vi "Pololu.Mgr - Get Status.vi"(8 "error in (no error)":errorcluster, 11 "PololuCtrl in":refnum<class "PololuCtrl.lvclass">) -> (0 "error out":errorcluster, 1 "Pos(Deg)":dbl[](array[numeric]), 2 "Moving":bool, 3 "PololuCtrl out":refnum<class "PololuCtrl.lvclass">)   [LabVIEW 2018, in "PololuCtrl.lvclass"]
uses:
  PololuCtrl.lvclass
  SubVIs/Pololu.Commands.ctl
  PololuCtrl.lvclass/PololuCtrl.ctl
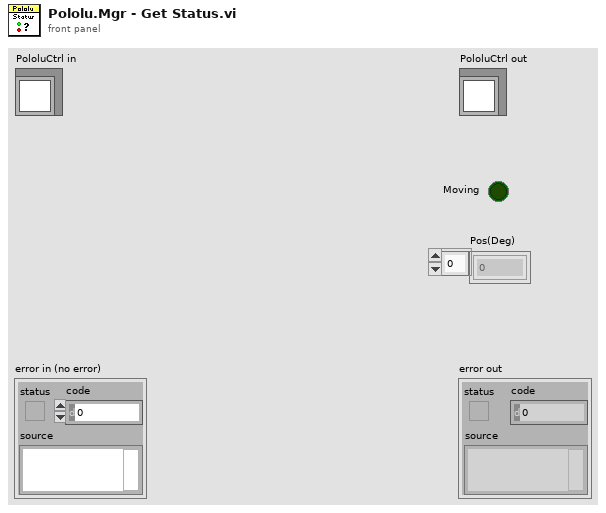
[diagram p1: front panel]
types:
  T1 = typedef "Pololu.Commands.ctl" = enum16{"Set Pos", "Set Speed", "Set Accel", "Get Pos", "Get Mov Status", "Get Errors"}
  T2 = typedef "Pololu.Device Config.ctl" = cluster{"Chan":u8, "Accel":u16, "Speed":u16, "Positions":dbl[], "Range Info":T3}
  T3 = typedef "Pololu.Device Range Config.ctl" = cluster{"Min us":dbl, "Max us":dbl, "Min deg":dbl, "Max deg":dbl, "LStopDeg":dbl, "UStopDeg":dbl}
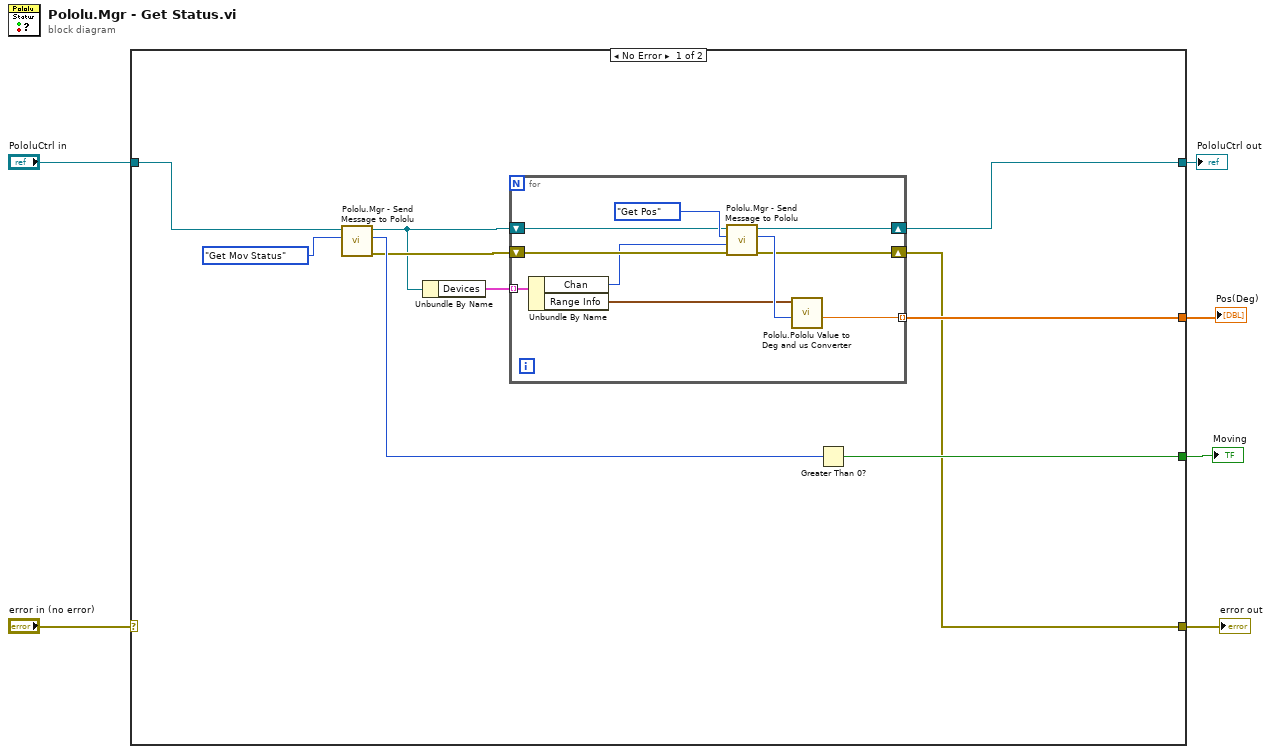
[diagram p0: block diagram]
diagram:
  n1 = case shown="No Error" "error in (no error)" {
    selector: "error in (no error)" -> [_ w28]
    tunnel: [w8 w28] -> w5
    tunnel: [w12 w27] -> w3
    tunnel: "PololuCtrl in" -> [w7 w27]
    tunnel: [w13 _] -> w2
    tunnel: [w9 _] -> w1
    frame No Error {
      n2 = call "Pololu.Mgr - Send Message to Pololu.vi"("Command"=Pololu.Commands."Get Mov Status", "PololuCtrl in"=w7) -> ("error out"=w14:errorcluster, "Response"=w15:u16, "PololuCtrl out"=w11:refnum<class "PololuCtrl.lvclass">)  [unwired: 7 in]
      n3 = Unbundle By Name(w11) -> ("Devices"=w10:T2[])
      n4 = for {
        shift-right: [w23] -> w12
        shift-left: w11 -> [w17]
        tunnel: w10 -> [w22] mode=indexing
        tunnel: [w19] -> w9 mode=indexing
        shift-right: [w18] -> w8
        shift-left: w14 -> [w26]
        n5 = Unbundle By Name(w22) -> ("Chan"=w21:u8, "Range Info"=w20:T3)
        n6 = call "Pololu.Mgr - Send Message to Pololu.vi"("error in (no error)"=w26, "Channel"=w21, "Command"=Pololu.Commands."Get Pos", "PololuCtrl in"=w17) -> ("error out"=w18:errorcluster, "Response"=w24:u16, "PololuCtrl out"=w23:refnum<class "PololuCtrl.lvclass">)  [unwired: 5 in]
        n7 = call "Pololu.Pololu Value to Deg and us Converter.vi"("Pololu Value"=w24, "Range Info"=w20) -> ("Pos (Deg)"=w19:dbl)  [unwired: 8 in, 1 out]
      }
      n8 = Greater Than 0?(x=w15) -> (x > 0?=w13:bool)
    }
    frame Error {
    }
  }
  "error out" <- w5
  "PololuCtrl out" <- w3
  "Moving" <- w2
  "Pos(Deg)" <- w1
